vi "Send CI-recieveStatus.vi"(7 "Message Priority (Normal)":T3=enum."Normal", 8 "error in (no error)":errorcluster, 10 "status":T1, 11 "Message Enqueuer":refnum<class "Message Enqueuer.lvclass">) -> (0 "error out":errorcluster, 3 "Message Enqueuer out":refnum<class "Message Enqueuer.lvclass">)   [LabVIEW 2020, in "CI-common_interface.lvlib" / "CI-recieveStatus Msg.lvclass"]
doc: "This VI sends the message to an actor."
uses:
  CI-recieveStatus Msg.lvclass
  <vilib>/ActorFramework/Message Enqueuer/Message Enqueuer.lvclass
  <vilib>/ActorFramework/Message Enqueuer/Message Priority.ctl
  CI-common_interface/CI-status_clust.ctl
  CI-common_interface/CI-module_enum.ctl
  C:/Program Files (x86)/National Instruments/LabVIEW 2020/vi.lib/ActorFramework/Message/Message.lvclass
  CI-recieveStatus Msg.lvclass/CI-recieveStatus Msg.ctl
  <vilib>/ActorFramework/Message Enqueuer/Message Enqueuer.lvclass/Message Enqueuer.ctl
  <vilib>/ActorFramework/Message Priority Queue/Priority Enqueue.vi
  CI-common_interface/CI-common_interface.lvclass
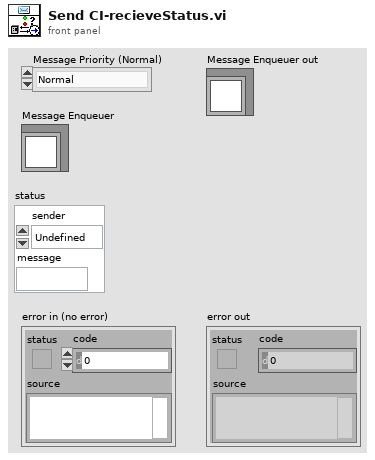
[diagram p1: front panel]
types:
  T1 = typedef "CI-common_interface.lvlib/CI-common_interface.lvclass/CI-status_clust.ctl" = cluster{"sender":T2, "message":string}
  T2 = typedef "CI-common_interface.lvlib/CI-common_interface.lvclass/CI-module_enum.ctl" = enum16{"Undefined", "HWM", "VDH", "GUI"}
  T3 = typedef "Actor Framework.lvlib/Message Enqueuer.lvclass/Message Priority.ctl" = enum16{"Low", "Normal", "High"}
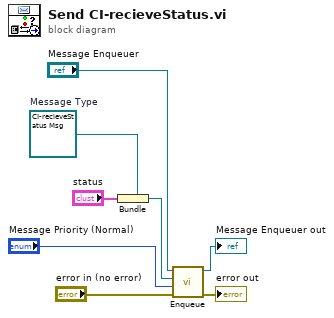
[diagram p0: block diagram]
diagram:
  w5 = refnum<class "CI-recieveStatus Msg.lvclass"> refnum  # Message Type
  n1 = Bundle(cluster=w5, "status") -> (w4:refnum<class "CI-recieveStatus Msg.lvclass">)
  n2 = call <vilib>:"Enqueue.vi"("error in (no error)"="error in (no error)", "Message Priority (Normal)"="Message Priority (Normal)", "Message"=w4, "Message Enqueuer in"="Message Enqueuer") -> ("error out"=→"error out":errorcluster, "Message Enqueuer out"=→"Message Enqueuer out":refnum<class "Message Enqueuer.lvclass">)  [unwired: 6 in]
